vi "Scale.vi"(8 "error in (no error)":errorcluster, 10 "Input":dbl, 11 "Meter in":refnum<class "Meter.lvclass">) -> (0 "error out":errorcluster, 2 "Output":dbl, 3 "Meter out":refnum<class "Meter.lvclass">)   [LabVIEW 2015, in "Meter.lvclass"]
uses:
  Meter.lvclass
  Mag Lab Properties/Mag Lab Parameters.lvclass
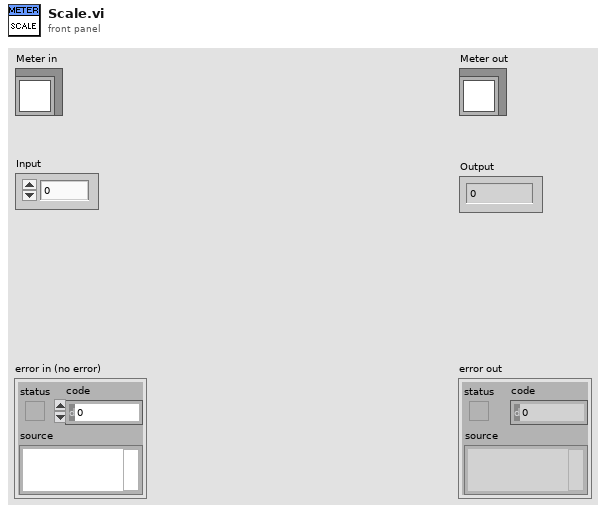
[diagram p1: front panel]
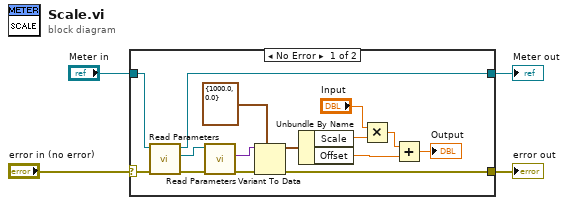
[diagram p0: block diagram]
diagram:
  n1 = case shown="No Error" "error in (no error)" {
    selector: "error in (no error)" -> [w12 w21]
    tunnel: [w11 w21] -> w3
    tunnel: [w10 w20] -> w1
    tunnel: "Meter in" -> [w13 w20]
    frame No Error {
      n2 = call-dynamic "Read Parameters.vi"("error in (no error)"=w12, "Mag Lab Root in"=w13) -> ("error out"=w16:errorcluster, "Mag Lab Parameters.lvclass"=w19:refnum<class "Mag Lab Parameters.lvclass">, "Mag Lab Root out"=w10:refnum<class "Meter.lvclass">)  [unwired: 7 in]
      n3 = call-dynamic "Read Parameters.vi"("error in (no error)"=w16, "Mag Lab Parameters in"=w19) -> ("error out"=w18:errorcluster, "Parameters"=w17:variant)  [unwired: 7 in, 1 out]
      n4 = Variant To Data(error in=w18, type=cluster{"Scale":dbl, "Offset":dbl} {"Scale"=1000.0, "Offset"=0.0} ("Parameters"), Variant=w17) -> (data=w14:cluster{"Scale":dbl, "Offset":dbl}, error out=w11:errorcluster)
      n5 = Unbundle By Name(w14) -> ("Scale"=w7:dbl, "Offset"=w9:dbl)
      n6 = Multiply(x="Input", y=w7) -> (x*y=w6:dbl)
      n7 = Add(x=w6, y=w9) -> (x+y=→"Output":dbl)
    }
    frame Error {
    }
  }
  "error out" <- w3
  "Meter out" <- w1
